vi "Modbus TCP_Init.vi"(8 "error in (no error)":errorcluster, 9 "Port":u16=502, 10 "Slave Address":string="localhost", 11 "object in":refnum<class "Modbus TCP.lvclass">) -> (0 "error out":errorcluster, 3 "object out":refnum<class "Modbus TCP.lvclass">)   [LabVIEW 2023, in "HardwareAbstractionLayer_LVOOP.lvlib" / "Modbus TCP.lvclass"]
uses:
  Modbus TCP.lvclass
  Modbus TCP.lvclass/Modbus TCP.ctl
  <vilib>/NI/Modbus Library/API/Wrapper/Create TCP Master.vi
  <vilib>/NI/Modbus Library/API/Wrapper/API Main.lvlib
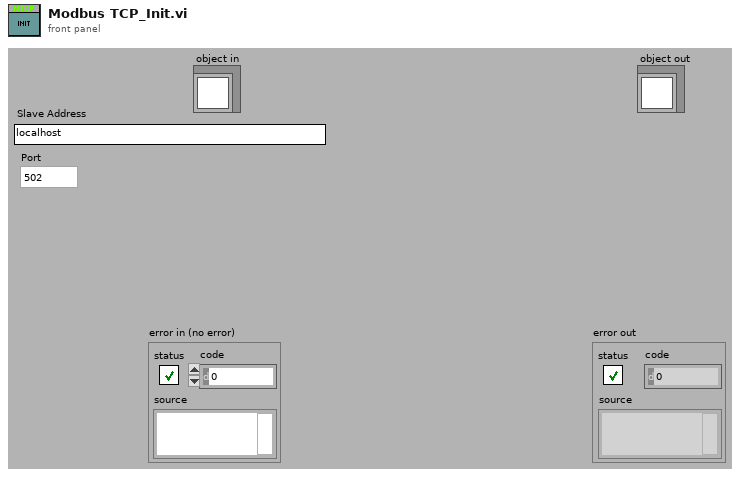
[diagram p1: front panel]
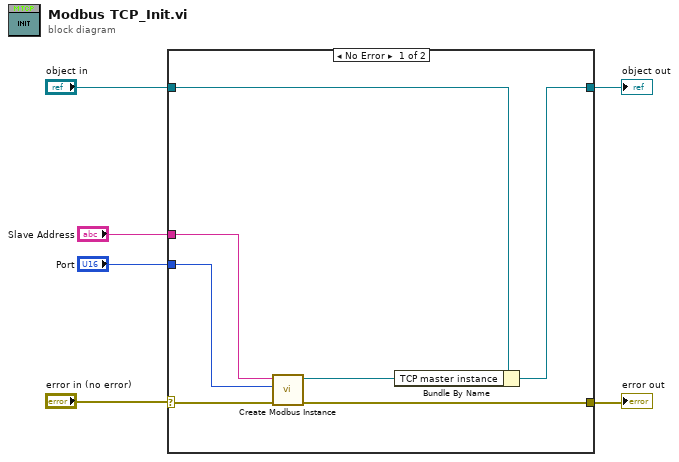
[diagram p0: block diagram]
diagram:
  n1 = case shown="No Error" "error in (no error)" {
    selector: "error in (no error)" -> [w11 w14]
    tunnel: "object in" -> [w13 w15]
    tunnel: [w12 w15] -> w5
    tunnel: [w10 w14] -> w3
    tunnel: "Slave Address" -> [w9 _]
    tunnel: "Port" -> [w8 _]
    frame No Error {
      n2 = call-poly <vilib>:"Create Modbus Instance.vi"("error in"=w11, "port (502)"=w8, "address"=w9) -> ("error out"=w10:errorcluster, "TCP master instance"=w7:refnum<class "Modbus Master.lvclass">)  [unwired: 7 in]
      n3 = Bundle By Name(cluster=w13, "TCP master instance"=w7) -> (w12:refnum<class "Modbus TCP.lvclass">)
    }
    frame Error {
    }
  }
  "object out" <- w5
  "error out" <- w3
